vi "Priority Enqueue.vi"(8 "error in (no error)":errorcluster, 9 "Message":refnum<class "Message.lvclass">, 10 "priority":i32, 11 "Priority Queue in":refnum<class "Message Priority Queue.lvclass">) -> (0 "error out":errorcluster, 3 "Priority Queue out":refnum<class "Message Priority Queue.lvclass">)   [LabVIEW 2020, in "Actor Framework.lvlib" / "Message Priority Queue.lvclass"]
uses:
  Message Priority Queue.lvclass
  Message/Message.lvclass
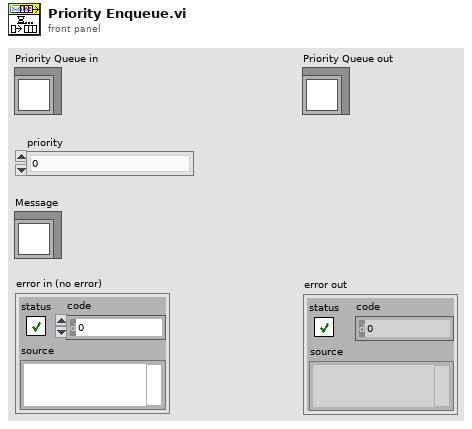
[diagram p1: front panel]
types:
  T1 = typedef "Actor Framework.lvlib/Message Priority Queue.lvclass/DVR Contents.ctl" = cluster{"# Waiting":u32, "Buffers":refnum<queue>[], "Wait Msg":refnum<queue>, "Wait Prior":refnum<queue>}
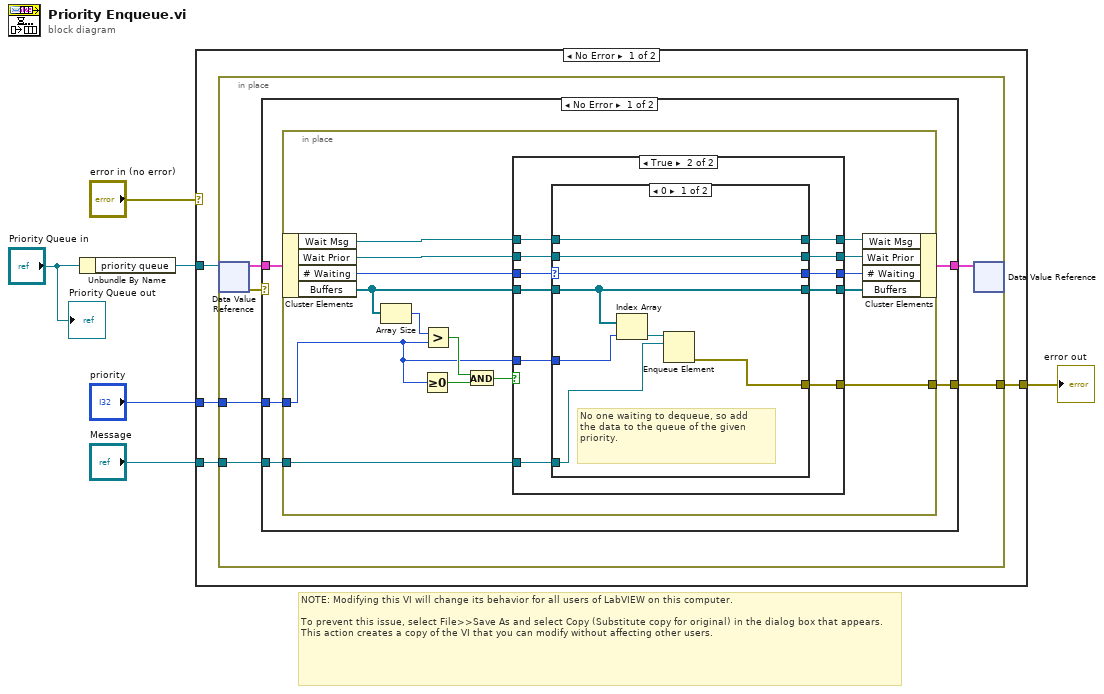
[diagram p0: block diagram]
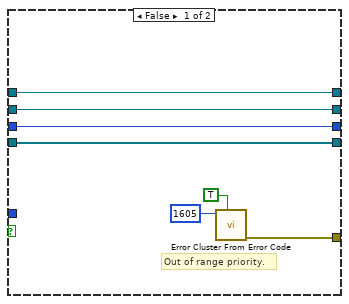
[diagram p2: hidden frame]
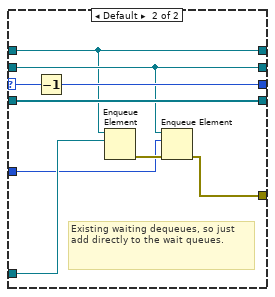
[diagram p3: hidden frame]
diagram:
  # "NOTE: Modifying this VI will change its behavior for all users of LabVIEW on this computer.\n\nTo prevent this issue, select File>>Save As and select Copy (Substitute copy for original) in the dialog box that appears. This action creates a copy of the VI that you can modify without affecting other users."
  n1 = Unbundle By Name("Priority Queue in") -> ("priority queue"=w2:refnum<data-value>)
  n2 = case shown="No Error" "error in (no error)" {
    selector: "error in (no error)" -> [_ w74]
    tunnel: [w9 w74] -> w5
    tunnel: w2 -> [w10 _]
    tunnel: "Message" -> [w8 _]
    tunnel: "priority" -> [w7 _]
    frame No Error {
      n3 = in-place {
        in-place-border: [w15] -> w9
        in-place-border: w8 -> [w12]
        in-place-border: w7 -> [w11]
        n4 = in-place-dvr #1(w10) -> (w13:T1, w16:errorcluster)
        n5 = case shown="No Error" w16 {
          selector: w16 -> [_ w73]
          tunnel: [w17 w73] -> w15
          tunnel: [w19 w72] -> w14
          tunnel: w13 -> [w21 w72]
          tunnel: w12 -> [w20 _]
          tunnel: w11 -> [w18 _]
          frame No Error {
            n6 = in-place {
              in-place-border: w20 -> [w36]
              in-place-border: w18 -> [w26]
              in-place-border: [w32] -> w17
              n7 = in-place-cluster #2(w21) -> ("Wait Msg"=w24:refnum<queue>, "Wait Prior"=w23:refnum<queue>, "# Waiting"=w34:u32, "Buffers"=w30:refnum<queue>[])
              n8 = Array Size(array=w30) -> (size(s)=w31:i32)
              n9 = Greater Or Equal To 0?(x=w26) -> (x >= 0?=w27:bool)
              n10 = Greater?(x=w31, y=w26) -> (0:w29:bool)
              n11 = And(x=w29, y=w27) -> (x .and. y?=w28:bool)
              n12 = case shown="True" w28 {
                tunnel: w30 -> [w43 w54]
                tunnel: w36 -> [_ w49]
                tunnel: [w43 w50] -> w35
                tunnel: w34 -> [w42 w53]
                tunnel: [w42 w52] -> w33
                tunnel: [w39 w48] -> w32
                tunnel: w26 -> [_ w51]
                tunnel: [w38 w47] -> w25
                tunnel: w24 -> [w38 w46]
                tunnel: w23 -> [w37 w45]
                tunnel: [w37 w44] -> w22
                frame False {
                  # "Out of range priority."
                  n13 = call <vilib>:"Error Cluster From Error Code.vi"("show call chain? (False)"=TRUE, "error code (0)"=1605) -> ("error out"=w39:errorcluster)  [unwired: 7 in]
                }
                frame True {
                  n14 = case shown="0" w53 {
                    selector: w53 -> [w62 w70]
                    tunnel: w54 -> [w59 w71]
                    tunnel: [w59 w71] -> w50
                    tunnel: [w62 w69] -> w52
                    tunnel: w51 -> [w60 w64]
                    tunnel: w49 -> [w58 w65]
                    tunnel: [w57 w63] -> w48
                    tunnel: [w56 w66] -> w47
                    tunnel: w46 -> [w56 w66]
                    tunnel: w45 -> [w55 w67]
                    tunnel: [w55 w67] -> w44
                    frame 0 {
                      # "No one waiting to dequeue, so add\nthe data to the queue of the given\npriority."
                      n15 = Index Array(array=w59, index=w60) -> (element=w61:refnum<queue>)
                      n16 = Enqueue Element(queue=w61, element=w58) -> (error out=w57:errorcluster)  [unwired: 2 in, 2 out]
                    }
                    frame Default {
                      # "Existing waiting dequeues, so just\nadd directly to the wait queues."
                      n17 = Decrement(x=w70) -> (x-1=w69:u32)
                      n18 = Enqueue Element(queue=w66, element=w65) -> (error out=w68:errorcluster)  [unwired: 2 in, 2 out]
                      n19 = Enqueue Element(queue=w67, element=w64, error in (no error)=w68) -> (error out=w63:errorcluster)  [unwired: 1 in, 2 out]
                    }
                  }
                }
              }
              n20 = in-place-cluster #2("Wait Msg"=w25, "Wait Prior"=w22, "# Waiting"=w33, "Buffers"=w35) -> (w19:T1)
            }
          }
          frame Error {
          }
        }
        n21 = in-place-dvr #1(w14) -> ()  [unwired: 2 out]
      }
    }
    frame Error {
    }
  }
  "error out" <- w5
  "Priority Queue out" <- "Priority Queue in"
